vi "Dashboard Main.vi"() -> ()   [LabVIEW 2018]
uses:
  <vilib>/Math Plots/2D Math Plots/2D Compass/2D Compass XCtrl/2D Compass.xctl
  <vilib>/Utility/miscctls.llb/LVRowAndColumnTypeDef.ctl
  <vilib>/event_ctls.llb/eventvkey.ctl
  <vilib>/Rock Robotics/Network Tables/NT Read Numeric Array.vi
  <vilib>/Rock Robotics/Network Tables/NT Write Numeric Array.vi
  <vilib>/Rock Robotics/WPI/Dashboard/WPI_DashboardLogging Global.vi
  <vilib>/Math Plots/2D Math Plots/2D Compass/2D Compass Datatype/2D Compass Datatype.lvclass
  <vilib>/Math Plots/2D Math Plots/2D Compass/2D Compass Datatype/Public/Plot Helper (Vector).vi
  <vilib>/Rock Robotics/Network Tables/NT Read Boolean Array.vi
panel:
  in  "Camera Settings Right":T1={"Frame Rate"=30, "Compression"=30, "Size"=1, "DB Camera Config"=FALSE} {"Frame Rate" scale=1.0..30.0; "Compression" scale=100.0..-1.0; "Size" items=["640x480", "320x240", "160x120"]}
  in  "Camera Name Right":string(combo)="No Camera Selection"
  out "Camera Perf":string
  in  "Camera Settings":T1={"Frame Rate"=30, "Compression"=30, "Size"=1, "DB Camera Config"=FALSE} {"Frame Rate" scale=1.0..30.0; "Compression" scale=100.0..-1.0; "Size" items=["640x480", "320x240", "160x120"]}
  in  "TCP":refnum<k5>
  in  "Rec Mode":enum32{"Stop", "Record", "Playback"}(radio)
  out "Robot IP":string
  out "Image Message":string="Timeout in Camera Communications"
  in  "Dashboard Tab":T2(tab)
  in  "Drive Type":string(combo)
  out "Reversed Modules":bool[](array[boolean])
  out "Front Right Swerve Module":refnum<class "2D Plot Datatype.lvclass">[](xcontrol) caption="2D Compass"
  out "NT Connection":bool
  out "Mode":T3(ring)=enum."Auto Disabled"
  out "Right Camera Perf":cluster{"Bandwidth (Mbps)":dbl, "FPS":dbl}
  in  "Write Swerve Offsets":bool
  out "Back Right Swerve Module":refnum<class "2D Plot Datatype.lvclass">[](xcontrol) caption="2D Compass"
  out "Back Left Swerve Module":refnum<class "2D Plot Datatype.lvclass">[](xcontrol) caption="2D Compass"
  out "Front Left Swerve Module":refnum<class "2D Plot Datatype.lvclass">[](xcontrol) caption="2D Compass"
  out "Scan Radar":picture
  out "Camera Image Right":T4(plugin-control)
  in  "Test Slider":dbl(slide) scale=0.0..100.0 scale format="%#_3g"
  in  "On/Off":bool caption="Solenoid"
  in  "Test Name":u16(ring) items=["Select the test to run..."]
  in  "Test Tree":string(tree)
  in  "Motor":cluster{"Value":dbl, "Enable":bool} {"Value" scale=-1.0..1.0 scale format="%#_3g"}
  out "Progress":T5 {"Test Progress" scale=0.0..100.0}
  in  "Rev/Fwd":cluster{"Forward":bool, "Reverse":bool}
  in  "Test Ring":u16(ring) items=["Monochrome", "Color"]
  out "Cmd Status":string
  in  "Execute Command":bool
  in  "Command Params":string[][](table)
  in  "Command Selection":i32(listbox)
  in  "CheckList":i32(listbox)
  out "Tree":string(tree)
  out "Camera Image":T4(plugin-control)
  out "Background":bool
  in  "Camera Name":string(combo)="No Camera Selection"
  # "HW"
  # "HW"
  # "Drive Options:"
  # "Swerve Vectors:"
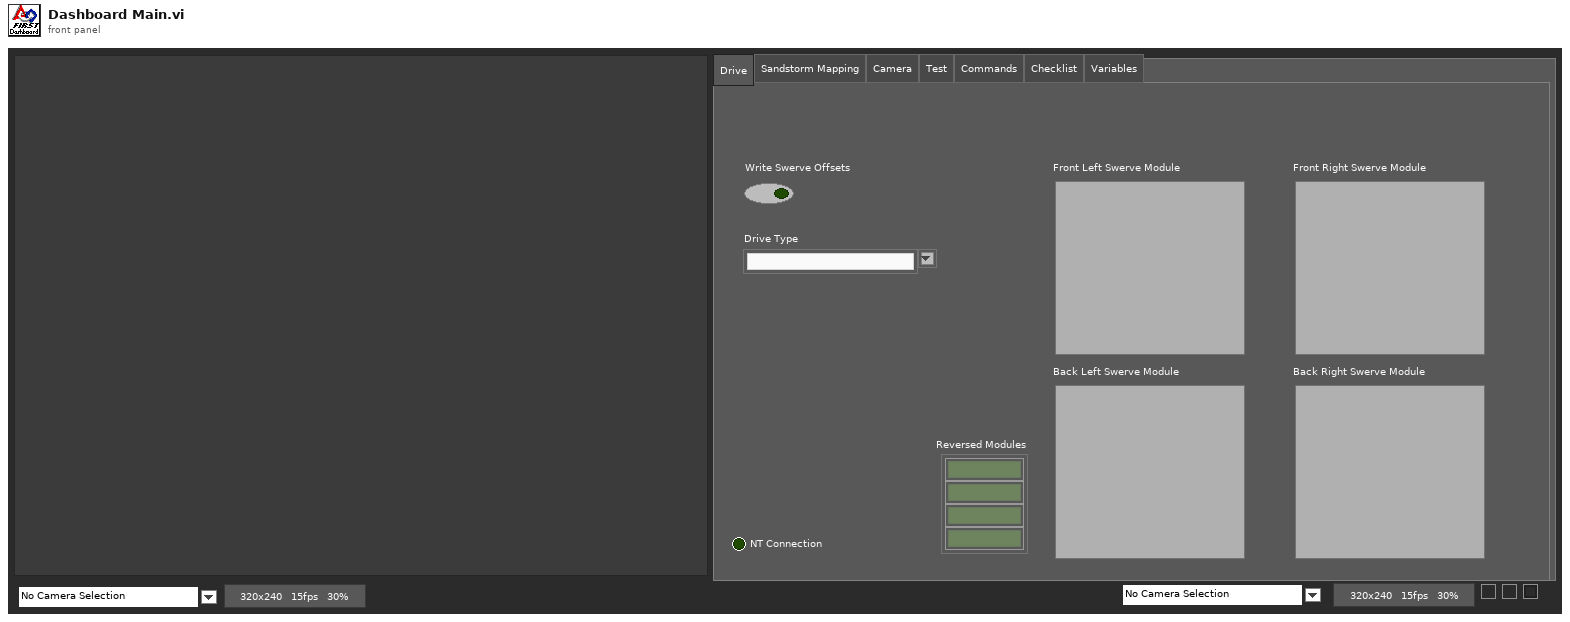
[diagram p1: front panel]
types:
  T1 = cluster{"Frame Rate":i32, "Compression":i32, "Size":u16, "DB Camera Config":bool}
  T2 = enum32{"Drive", "Sandstorm Mapping", "Camera", "Test", "Commands", "Checklist", "Variables"}
  T3 = enum8{"Tele-Op Disabled", "Tele-Op Enabled", "Auto Disabled", "Auto Enabled", "Test Disabled", "Test Enabled", "Disconnected", "No Code", "E-Stop"}
  T4 = typedef "IMAQ Image.ctl" = refnum<image>
  T5 = cluster{"Test Progress":u8, "Test Progress Text":string}
  T6 = cluster{"Save Path":path, "Interval (s)":dbl, "Keep":i32}
  T7 = enum32{"Drive", "Camera", "Basic", "Custom", "Test", "Commands", "Checklist", "Variables"}
  T8 = typedef "Image Type" = u32
  T9 = cluster{"IDs":cluster{"RPC field ID":u16, "Unique ID":u16}, "String":string}
  T10 = enum16{"open", "replace", "create", "open or create", "replace or create", "replace or create with confirmation"}
  T11 = cluster{"Error Strings":string, "Disable Counts":cluster{u16, u16}, "Rail Faults":cluster{u16, u16, u16}, "Robot IP":string, "DB Mode":u8, "Event Info":cluster{"Name":string, "Type":u8, "Number":u16, "Replay":u8}}
  T12 = cluster{"Storage":cluster{"Disk Free":u64, "RAM Block":u32, "RAM free":u32}, "CPU Utilization":cluster{"CPU % ISR":sgl, "CPU % Time Crit":sgl, "CPU % Timed Str":sgl, "CPU % High":sgl, "CPU % Above":sgl, "CPU % Normal":sgl, "CPU % Low":sgl}, "CAN":cluster{"% Bus Utilization":sgl, "Bus Off Cnt":u32, "TX_FIFO Full Cnt":u32, "Receive Error Cnt":u8, "Transmit Error Cnt":u8}, "HID":cluster{"HID Outputs":u32, "Rumble Low":u16, "Rumble High":u16}[]}
  T13 = cluster{"Status bits":cluster{"Test Mode":bool, "Autonomous":bool, "Enabled":bool, "Code Start":bool, "Brownout":bool, "Reserved 2":bool, "Reserved 3":bool, "E-Stop":bool}, "Code Trace":cluster{"Disabled":bool, "TeleOp":bool, "Auto":bool, "Test":bool}, "Controller Type":enum16{"unknown", "cRIO", "roboRio"}, "Code?":enum16{"unknown", "noCode", "code"}, "Battery V":dbl}
  T14 = cluster{"Control Bits":cluster{"TestMode":bool, "Autonomous":bool, "Enabled":bool, "FMS Present":bool, bool, bool, bool, "E-Stop":bool}, "Team Station ":u8, "Countdown":sgl, "Joystick Values":cluster{"Axes":dbl[], "Buttons":bool[], "POVs":i16[]}[]}
  T15 = cluster{"Axes":dbl[], "Buttons":bool[], "POVs":i16[]}[]
  T16 = cluster{"Axes":dbl[], "Buttons":bool[], "POVs":i16[]}
  T17 = typedef "LVBoundsTypeDef.ctl" = cluster{"Width":u32, "Height":u32}
  T18 = cluster{"Camera Image":refnum<vi>, "Dashboard Tab":refnum<vi>, "Background":refnum<vi>, "Rec Mode":refnum<vi>, "Test Slider":refnum<vi>, "On/Off ":refnum<vi>, "Test Ring":refnum<vi>, "Rev/Fwd":refnum<vi>, "Test Name":refnum<vi>, "Motor":refnum<vi>, "Progress":refnum<vi>, "CheckList":refnum<vi>, "Tree":refnum<vi>, "Test Tree":refnum<vi>, "Command Params":refnum<vi>, "Command Selection":refnum<vi>, "Execute Command":refnum<vi>, "Cmd Status":refnum<vi>, "Camera Settings":refnum<vi>, "Camera Name":refnum<vi>, "Camera Perf":refnum<vi>, "Camera Settings Right":refnum<vi>, "Camera Name Right":refnum<vi>, "Camera Image Right":refnum<vi>}
  T19 = cluster{"Global Rectangle":i32[], "Contours":cluster{"Contour Type":u32, "ROI Type":u32, "Points":i32[]}[]}
  T20 = cluster{"Camera Name":string, string, "Saved DB Images Info":cluster{"Save Path":path, "Interval (s)":dbl, "Keep":i32}}
  T21 = cluster{"Camera Name Right":string, string, "Saved DB Images Info":cluster{"Save Path":path, "Interval (s)":dbl, "Keep":i32}}
  T22 = cluster{"Operation":enum16{"Update", "Clear"}, "Color Box":u32}[]
  T23 = typedef "eventvkey.ctl" = enum16{"ASCII", "Enter", "Return", "Shift", "Ctrl", "Alt", "Cmd", "Opt", "Caps", "NumLock", "Clear", "Break", "Up", "Down", "Left", "Right", "Insert", "Delete", "Home", "End", "PageUp", "PageDown", "Escape", "Help", "Pause", "ScrollLock", "F1", "F2", "F3", "F4", "F5", "F6", "F7", "F8", "F9", "F10", "F11", "F12", "F13", "F14", "F15", "F16", "F17", "F18", "F19", "F20", "F21", "F22", "F23", "F24", "Play", "VolumeUp", "VolumeDown", "Mute", "Two Byte Char"}
  T24 = cluster{"Image Size":bool, "Image Type":bool, "Pixel Value":bool, "ROI Information":bool, "Zoom Factor":bool}
  T25 = cluster{"Operation":enum16{"Update", "Clear"}, "Color Box":u32}
  T26 = typedef "LVRowAndColumnTypeDef.ctl" = cluster{"Row":i32, "Column":i32}
  T27 = cluster{"Shift":bool, "Ctrl":bool, "Alt":bool, "Cmd":bool, "Opt":bool}
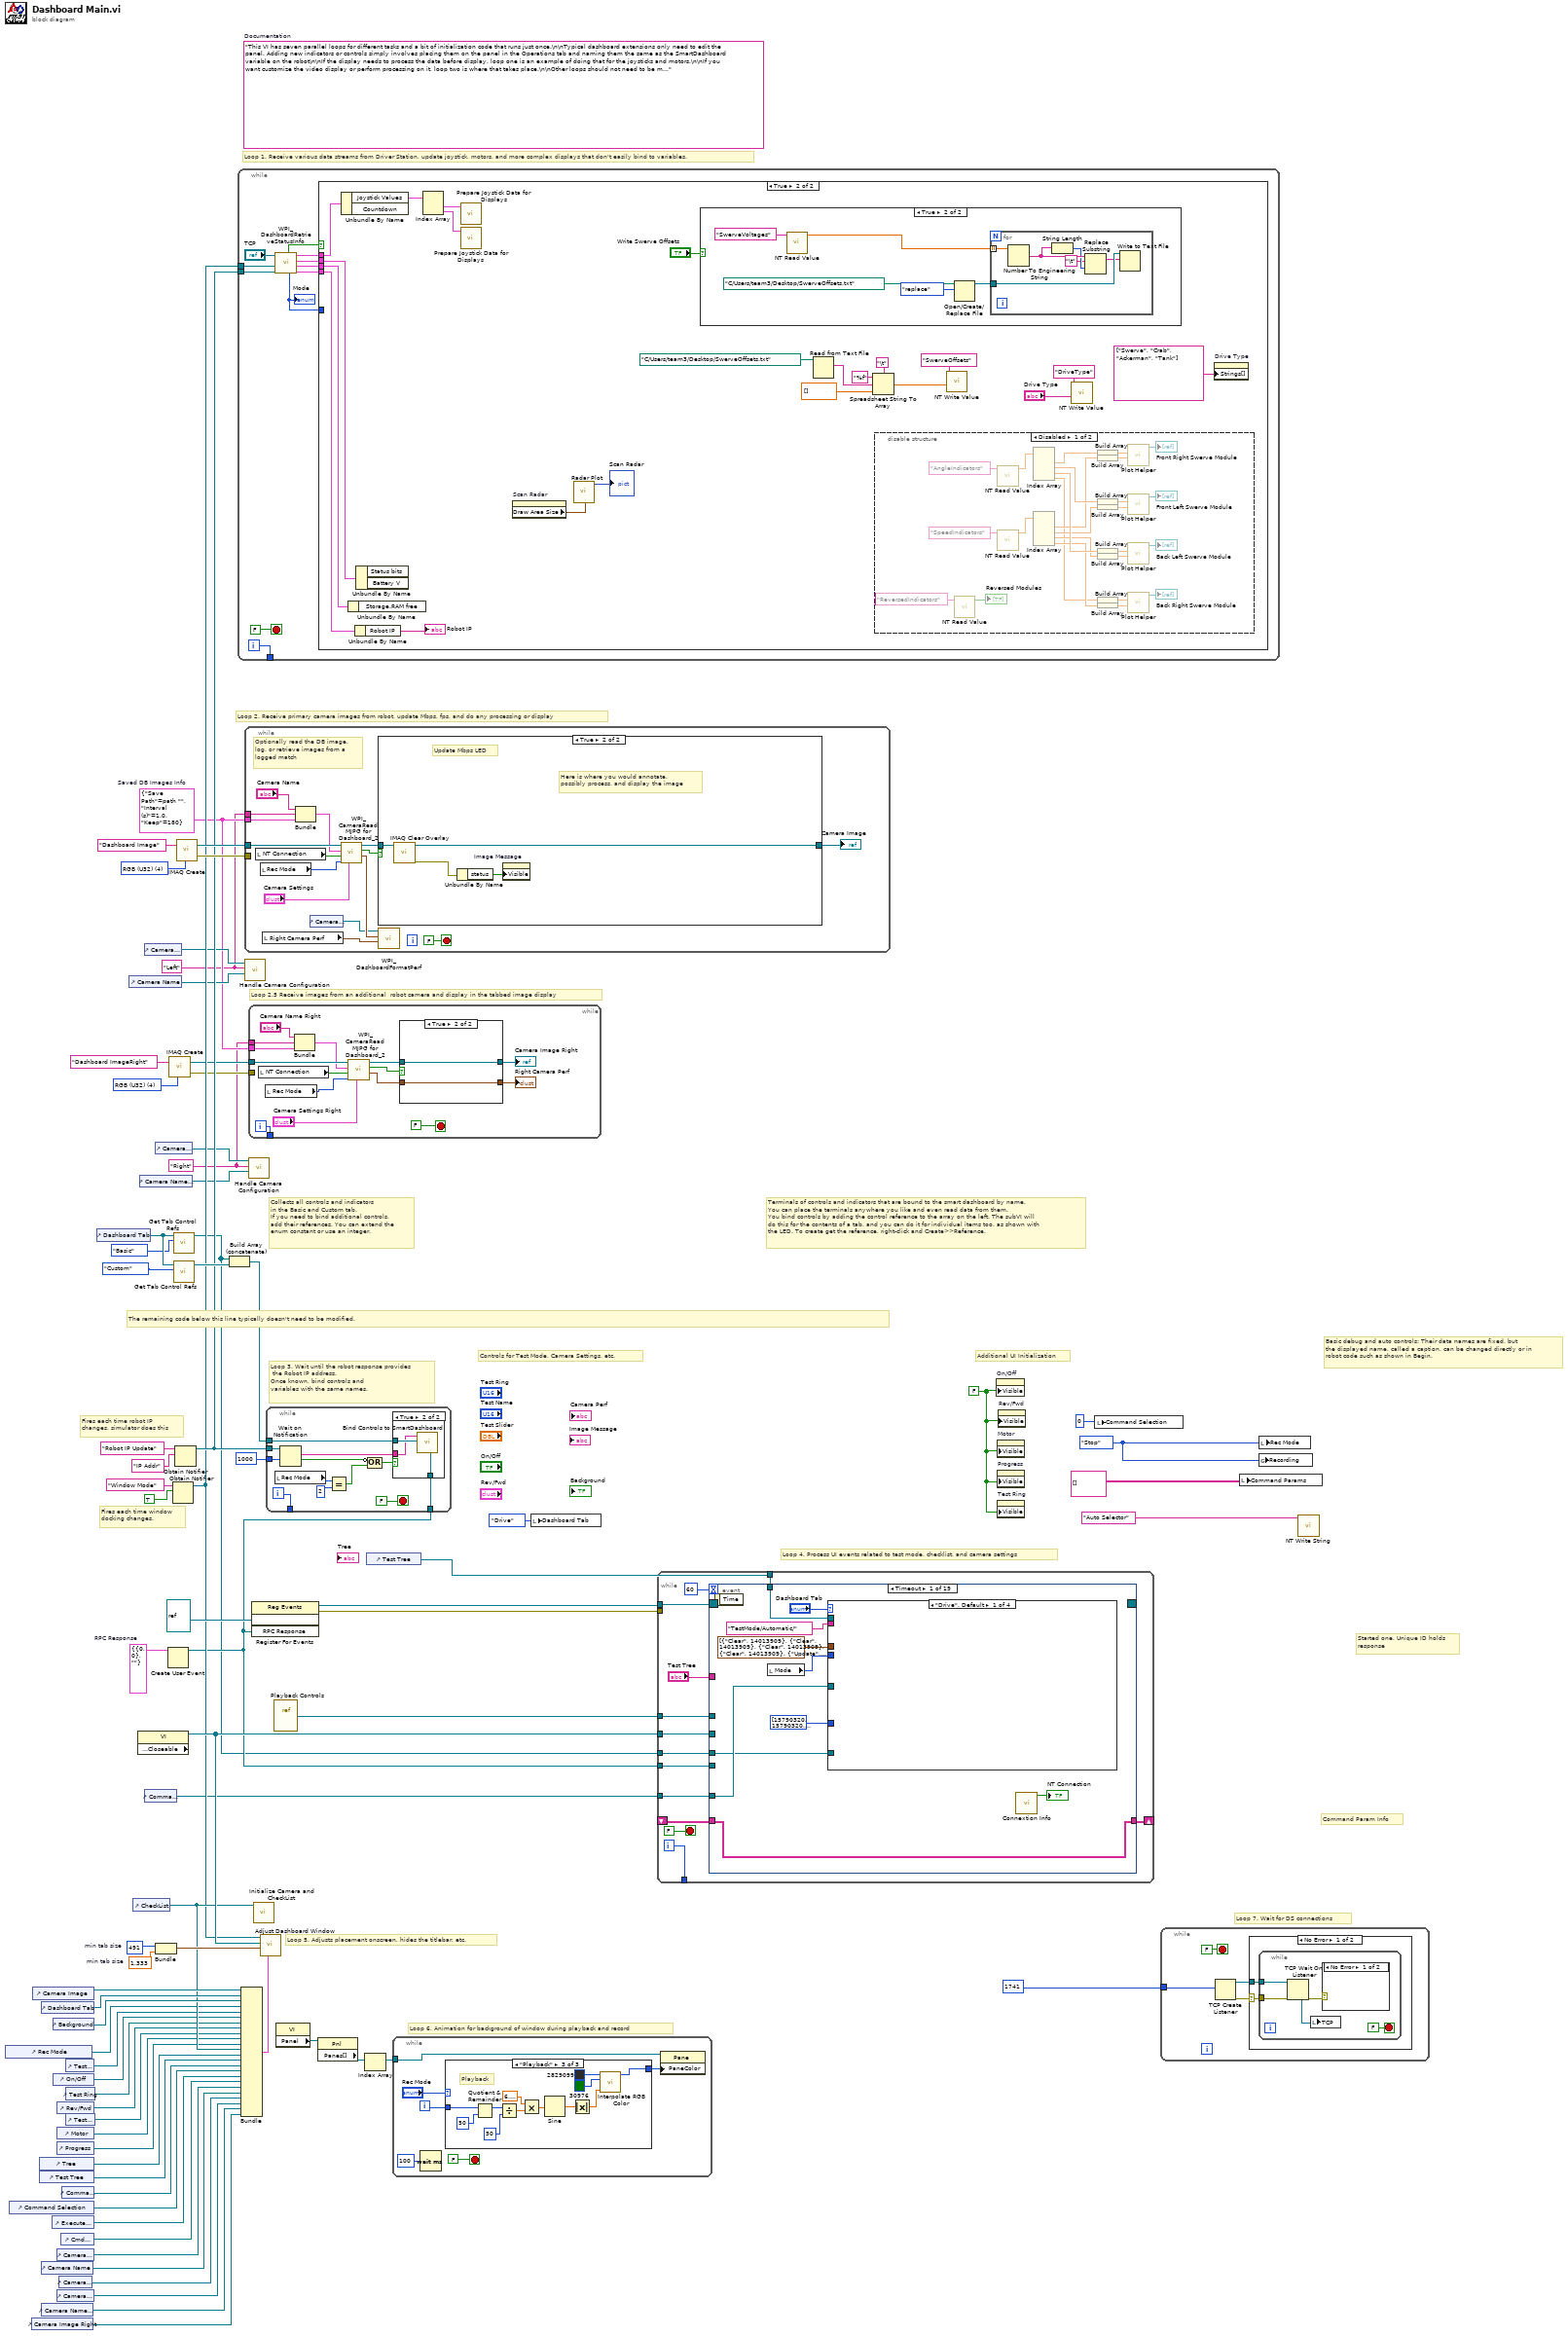
[diagram p0: block diagram]
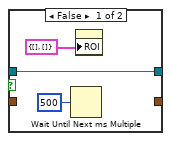
[diagram p2: hidden frame]
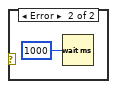
[diagram p3: hidden frame]
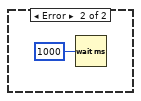
[diagram p4: hidden frame]
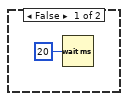
[diagram p5: hidden frame]
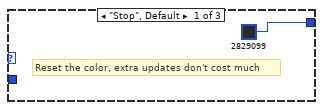
[diagram p8: hidden frame]
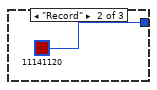
[diagram p9: hidden frame]
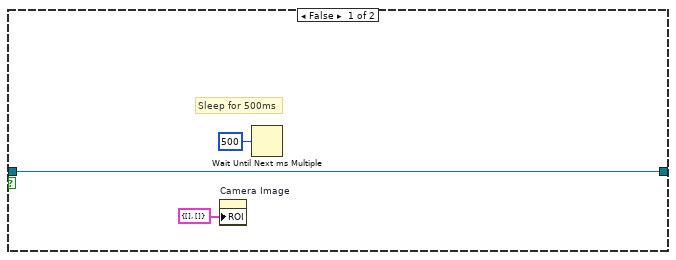
[diagram p11: hidden frame]
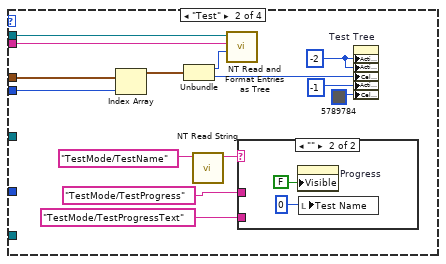
[diagram p12: hidden frame]
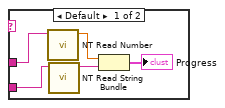
[diagram p13: hidden frame]
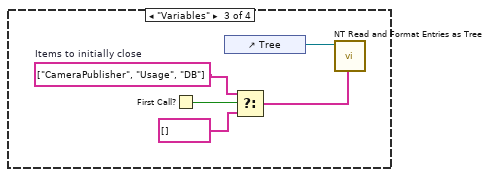
[diagram p14: hidden frame]
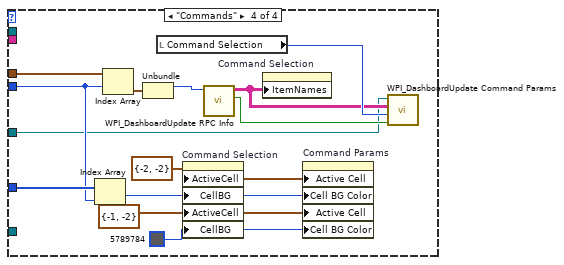
[diagram p15: hidden frame]
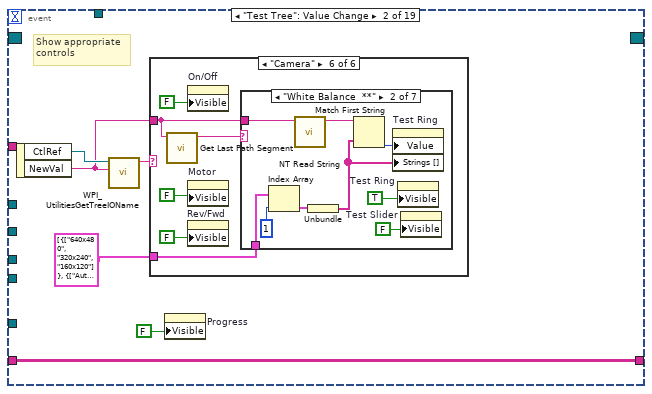
[diagram p16: hidden frame]
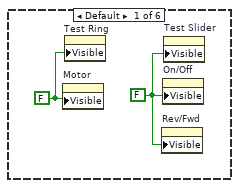
[diagram p17: hidden frame]
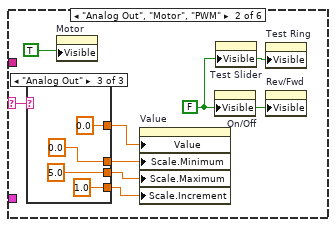
[diagram p18: hidden frame]
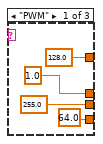
[diagram p19: hidden frame]
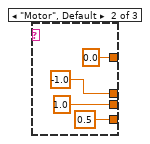
[diagram p20: hidden frame]
diagram:
  w4 = T6 {"Save Path"=path "", "Interval (s)"=1.0, "Keep"=180}  # Saved DB Images Info
  w3 = "Right"
  w2 = "Left"
  w14 = T8 4 items=["Grayscale (U8)", "Grayscale (I16)", "Grayscale (SGL)", "Complex (CSG)", "RGB (U32)", "HSL (U32)", "RGB (U64)"] ("Image Type")
  w29 = T9 {"IDs"={"RPC field ID"=0, "Unique ID"=0}, "String"=""}  # RPC Response
  w51 = 491  # min tab size
  w50 = 1.333  # min tab size
  w58 = enum32{"Stop", "Record", "Playback"}."Stop" ("Rec Mode")
  w35 = FALSE ("Visible")
  (unwired) "This VI has seven parallel loops for different tasks and a bit of initialization code that runs just once.\n\nTypical dashboard extensions only need to edit the panel. Adding new indicators or controls simply involves placing them on the panel in the Operations tab and naming them the same as the SmartDashboard variable on the robot\n\nIf the display needs to process the data before display, loop one is an example of doing that for the joysticks and motors.\n\nIf you want customize the video display or perform processing on it, loop two is where that takes place.\n\nOther loops should not need to be modified. They are pretty standard, and document the task they perform."  # Documentation
  w75 = T8 4 items=["Grayscale (U8)", "Grayscale (I16)", "Grayscale (SGL)", "Complex (CSG)", "RGB (U32)", "HSL (U32)", "RGB (U64)"] ("Image Type")
  # "Loop 2.5 Receive images from an additional  robot camera and display in the tabbed image display"
  # "Command Param Info"
  # "Started one, Unique ID holds\nresponse"
  # "Loop 7. Wait for DS connections"
  # "Basic debug and auto controls: Their data names are fixed, but\nthe displayed name, called a caption, can be changed directly or in\nrobot code such as shown in Begin."
  # "Controls for Test Mode, Camera Settings, etc."
  # "Additional UI Initialization"
  # "Loop 6. Animation for background of window during playback and record"
  # "Fires each time robot IP\nchanges, simulator does this"
  # "Fires each time window\ndocking changes."
  # "Collects all controls and indicators\nin the Basic and Custom tab.\nIf you need to bind additional controls,\nadd their references. You can extend the\nenum constant or use an integer."
  # "The remaining code below this line typically doesn't need to be modified."
  # "Loop 4. Process UI events related to test mode, checklist, and camera settings"
  # "Terminals of controls and indicators that are bound to the smart dashboard by name.\nYou can place the terminals anywhere you like and even read data from them.\nYou bind controls by adding the control reference to the array on the left. The subVI will\ndo this for the contents of a tab, and you can do it for individual items too, as shown with\nthe LED. To create get the reference, right-click and Create>>Reference."
  # "Loop 3. Wait until the robot response provides\n the Robot IP address.\nOnce known, bind controls and\nvariables with the same names."
  # "Loop 5. Adjusts placement onscreen, hides the titlebar, etc."
  # "Loop 1. Receive various data streams from Driver Station, update joystick, motors, and more complex displays that don't easily bind to variables."
  # "Loop 2. Receive primary camera images from robot, update Mbps, fps, and do any processing or display"
  n1 = control-ref of="Rec Mode"() -> (w41:refnum<vi>)
  n2 = control-ref of="Command Selection"() -> (w28:refnum<vi>)
  n3 = control-ref of="Camera Image Right"() -> (w7:refnum<vi>)
  n4 = control-ref of="Camera Image"() -> (w53:refnum<vi>)
  n5 = control-ref of="Tree"() -> (w45:refnum<vi>)
  n6 = control-ref of="Test Tree"() -> (w44:refnum<vi>)
  n7 = control-ref of="Dashboard Tab"() -> (w52:refnum<vi>)
  n8 = control-ref of="Camera Name"() -> (w19:refnum<vi>)
  n9 = control-ref of="Camera Name Right"() -> (w8:refnum<vi>)
  n10 = control-ref of="Execute Command"() -> (w30:refnum<vi>)
  n11 = control-ref of="Background"() -> (w48:refnum<vi>)
  n12 = control-ref of="On/Off"() -> (w39:refnum<vi>)
  n13 = control-ref of="Progress"() -> (w36:refnum<vi>)
  n14 = control-ref of="Camera Settings"() -> (w20:refnum<vi>)
  n15 = control-ref of="Camera Settings Right"() -> (w9:refnum<vi>)
  n16 = control-ref of="Rev/Fwd"() -> (w37:refnum<vi>)
  n17 = control-ref of="Motor"() -> (w42:refnum<vi>)
  n18 = control-ref of="Camera Perf"() -> (w18:refnum<vi>)
  n19 = control-ref of="Cmd Status"() -> (w24:refnum<vi>)
  n20 = control-ref of="Command Params"() -> (w31:refnum<vi>)
  n21 = control-ref of="Test Slider"() -> (w40:refnum<vi>)
  n22 = control-ref of="Test Ring"() -> (w38:refnum<vi>)
  n23 = control-ref of="Test Name"() -> (w43:refnum<vi>)
  n24 = control-ref of="Dashboard Tab"() -> (w56:refnum<vi>)
  n25 = control-ref of="Camera Name"() -> (w21:refnum<vi>)
  n26 = control-ref of="CheckList"() -> (w46:refnum<vi>)
  n27 = property class="VI" props=["Front Panel.Closeable"]() -> (reference out=w57:refnum<vi>)  [unwired: 2 in, 2 out]
  n28 = control-ref of="Camera Name Right"() -> (w10:refnum<vi>)
  n29 = control-ref of="Camera Settings"() -> (w22:refnum<vi>)
  n30 = control-ref of="Command Params"() -> (w23:refnum<vi>)
  n31 = control-ref of="Camera Settings Right"() -> (w11:refnum<vi>)
  n32 = Bundle("min tab size"=w51, "min tab size"=w50) -> (w49:cluster{"min tab size":i32, "min tab size":dbl})  [unwired: 1 in]
  n33 = Create User Event(user event datatype=w29) -> (user event=w25:refnum<user-event>)  [unwired: 1 in, 1 out]
  n34 = call "IMAQ Create"("Image Name"="Dashboard ImageRight", "Image Type"=w14) -> ("New Image"=w13:T4, "error out"=w12:errorcluster)  [unwired: 2 in, 1 out]
  n35 = Obtain Notifier(name (unnamed)="Window Mode", notification data type=TRUE) -> (notifier out=w33:refnum<notifier>)  [unwired: 2 in, 2 out]
  n36 = call <vilib>:"Get Tab Control Refs.vi"("Page Index"=T7."Basic" ("Dashboard Tab"), "TabControl in"=w56) -> ("ControlsOnPage"=w17:refnum<vi>[])  [unwired: 9 in]
  n37 = call <vilib>:"Get Tab Control Refs.vi"("Page Index"=T7."Custom" ("Dashboard Tab"), "TabControl in"=w56) -> ("ControlsOnPage"=w55:refnum<vi>[])  [unwired: 9 in]
  n38 = Obtain Notifier(name (unnamed)="Robot IP Update", notification data type="IP Addr" ("name (unnamed)")) -> (notifier out=w34:refnum<notifier>)  [unwired: 2 in, 2 out]
  n39 = call "IMAQ Create"("Image Name"="Dashboard Image", "Image Type"=w75) -> ("New Image"=w73:T4, "error out"=w72:errorcluster)  [unwired: 2 in, 1 out]
  n40 = Build Array (concatenate)(w17, w55) -> (w54:refnum<vi>[])
  n41 = while {
    tunnel: [w85] -> _
    tunnel: w34 -> [w79]
    tunnel: w33 -> [w76]
    i -> [w85]
    stop <- FALSE stop-if-true
    n42 = call <vilib>:"WPI_DashboardRetrieveStatusInfo.vi"("Binding Refnum"=w79, "Window Mode Notifier"=w76, "TCP Cnx"="TCP") -> ("Power and Errors"=w80:T11, "Robot Metrics"=w83:T12, "Status Info"=w84:T13, "Control Info"=w81:T14, "Robot Mode"=w78:T3, "Process?"=w82:bool)  [unwired: 3 in]
    "Mode" <- w78
    n43 = case shown="True" w82 {
      tunnel: w84 -> [_ w108]
      tunnel: w83 -> [_ w107]
      tunnel: w81 -> [_ w106]
      tunnel: w80 -> [_ w105]
      tunnel: w78 -> [_ _]
      frame False {
        n44 = Wait (ms)(milliseconds to wait=u32 20) -> ()  [unwired: 1 out]
      }
      frame True {
        n45 = Unbundle By Name(w106) -> ("Joystick Values"=w99:T15)  [unwired: 1 out]
        n46 = Unbundle By Name(w107) -> ()  [unwired: 1 out]
        n47 = Unbundle By Name(w105) -> ("Robot IP"=→"Robot IP":string)
        n48 = Unbundle By Name(w108) -> ()  [unwired: 2 out]
        n49 = Index Array(array=w99) -> (element #1=w104:T16, element #2=w103:T16)  [unwired: 2 in]
        n50 = call "Prepare Joystick Data for Displays.vi"("Joystick Values"=w104) -> ()  [unwired: 8 in, 3 out]
        n51 = call "Prepare Joystick Data for Displays.vi"("Joystick Values"=w103) -> ()  [unwired: 8 in, 3 out]
        n52 = property on="Scan Radar" class="Pict"() -> ("Draw Area Size"=w97:T17)  [unwired: 2 in, 2 out]
        n53 = call <vilib>:"Radar Plot.vi"("dimension (w,h)"=w97) -> ("new picture"=→"Scan Radar":picture)  [unwired: 14 in]
        n54 = case shown="True" "Write Swerve Offsets" {
          frame False {
          }
          frame True {
            n55 = call-poly <vilib>:"NT Read Value.vi"("Name"="SwerveVoltages") -> ("Numeric Array"=w135:dbl[])  [unwired: 9 in, 1 out]
            n56 = Open/Create/Replace File(file path (use dialog)=path "C:/Users/team3/Desktop/SwerveOffsets.txt" ("file (use dialog)"), operation (0:open)=T10."replace") -> (refnum out=w138:refnum<file>)  [unwired: 4 in, 2 out]
            n57 = for {
              tunnel: w138 -> [w144]
              tunnel: w135 -> [w145] mode=indexing
              n58 = Number To Engineering String(4:w145) -> (0:w143:string)  [unwired: 3 in]
              n59 = String Length(string=w143) -> (length=w142:i32)
              n60 = Replace Substring(3:w142, 4:"\t", 5:w143) -> (1:w140:string)  [unwired: 1 in, 1 out]
              n61 = Write to Text File(file (use dialog)=w144, text=w140) -> ()  [unwired: 2 in, 3 out]
            }
          }
        }
        n62 = Read from Text File(file (use dialog)=path "C:/Users/team3/Desktop/SwerveOffsets.txt") -> (text=w92:string)  [unwired: 3 in, 3 out]
        n63 = Spreadsheet String To Array(delimiter (Tab)="\t", format string="%f", spreadsheet string=w92, array type (2D Dbl)=dbl[] []) -> (array=w91:dbl[])
        n64 = disable-structure shown="Disabled" {
          frame Disabled {
            n65 = call-poly <vilib>:"NT Read Value.vi"("Name"="ReversedIndicators") -> ("Boolean Array"=→"Reversed Modules":bool[])  [unwired: 9 in, 1 out]
            n66 = call-poly <vilib>:"NT Read Value.vi"("Name"="AngleIndicators") -> ("Numeric Array"=w127:dbl[])  [unwired: 9 in, 1 out]
            n67 = call-poly <vilib>:"NT Read Value.vi"("Name"="SpeedIndicators") -> ("Numeric Array"=w126:dbl[])  [unwired: 9 in, 1 out]
            n68 = Index Array(array=w127) -> (element #1=w122:dbl, element #2=w121:dbl, element #3=w120:dbl, element #4=w109:dbl)  [unwired: 4 in]
            n69 = Index Array(array=w126) -> (element #1=w117:dbl, element #2=w114:dbl, element #3=w112:dbl, element #4=w110:dbl)  [unwired: 4 in]
            n70 = Build Array(w122) -> (w124:dbl[])
            n71 = Build Array(w117) -> (w116:dbl[])
            n72 = Build Array(w121) -> (w123:dbl[])
            n73 = Build Array(w114) -> (w115:dbl[])
            n74 = Build Array(w120) -> (w119:dbl[])
            n75 = Build Array(w112) -> (w113:dbl[])
            n76 = Build Array(w109) -> (w118:dbl[])
            n77 = Build Array(w110) -> (w111:dbl[])
            n78 = call-poly <vilib>:"Plot Helper.vi"("radius vector"=w116, "theta vector"=w124) -> ("2D Plot Class Obj Array out"=→"Front Right Swerve Module":refnum<class "2D Plot Datatype.lvclass">[])  [unwired: 2 in, 7 out]
            n79 = call-poly <vilib>:"Plot Helper.vi"("radius vector"=w115, "theta vector"=w123) -> ("2D Plot Class Obj Array out"=→"Front Left Swerve Module":refnum<class "2D Plot Datatype.lvclass">[])  [unwired: 2 in, 7 out]
            n80 = call-poly <vilib>:"Plot Helper.vi"("radius vector"=w113, "theta vector"=w119) -> ("2D Plot Class Obj Array out"=→"Back Left Swerve Module":refnum<class "2D Plot Datatype.lvclass">[])  [unwired: 2 in, 7 out]
            n81 = call-poly <vilib>:"Plot Helper.vi"("radius vector"=w111, "theta vector"=w118) -> ("2D Plot Class Obj Array out"=→"Back Right Swerve Module":refnum<class "2D Plot Datatype.lvclass">[])  [unwired: 2 in, 7 out]
          }
          frame Enabled {
          }
        }
        n82 = call-poly <vilib>:"NT Write Value.vi"("Numeric Array"=w91, "Name"="SwerveOffsets") -> ()  [unwired: 9 in, 1 out]
        n83 = call-poly <vilib>:"NT Write Value.vi"("String"="Drive Type", "Name"="DriveType") -> ()  [unwired: 9 in, 1 out]
        n84 = property on="Drive Type" class="CmbBox"("Strings[]"=string[] ["Swerve", "Crab", "Ackerman", "Tank"] ("Strings []")) -> ()  [unwired: 2 in, 2 out]
      }
    }
  }
  n85 = Bundle("Camera Image"=w53, "Dashboard Tab"=w52, "Background"=w48, "Rec Mode"=w41, "Test Slider"=w40, "On/Off"=w39, "Test Ring"=w38, "Rev/Fwd"=w37, "Test Name"=w43, "Motor"=w42, "Progress"=w36, "CheckList"=w46, "Tree"=w45, "Test Tree"=w44, "Command Params"=w31, "Command Selection"=w28, "Execute Command"=w30, "Cmd Status"=w24, "Camera Settings"=w20, "Camera Name"=w19, "Camera Perf"=w18, "Camera Settings Right"=w9, "Camera Name Right"=w8, "Camera Image Right"=w7) -> (w47:T18)  [unwired: 1 in]
  n86 = call "Handle Camera Configuration.vi"("CameraNameRef"=w21, "Display Name"=w2, "ClusterRef"=w22) -> ()  [unwired: 9 in]
  n87 = while {
    tunnel: w73 -> [w159]
    tunnel: w72 -> [_]
    tunnel: w4 -> [w152]
    tunnel: w2 -> [w149]
    stop <- FALSE stop-if-true
    # "Optionally read the DB image,\nlog, or retrieve images from a\nlogged match"
    n88 = local read "NT Connection"() -> (w153:bool)
    n89 = local read "Rec Mode"() -> (w156:enum32{"Stop", "Record", "Playback"})
    n90 = local read "Right Camera Perf"() -> (w147:cluster{"Bandwidth (Mbps)":dbl, "FPS":dbl})
    n91 = Bundle("Camera Name"="Camera Name", w149, "Saved DB Images Info"=w152) -> (w151:T20)  [unwired: 1 in]
    n92 = control-ref of="Camera Perf"() -> (w146:refnum<vi>)
    n93 = call <vilib>:"WPI_CameraRead MJPG for Dashboard_2.vi"("Camera Settings"="Camera Settings", "Rec Mode"=w156, "NT Connection"=w153, "Capture Info"=w151, "Image in"=w159) -> ("perf info"=w148:cluster{"Bandwidth (Mbps)":dbl, "fps":dbl}, "Active"=w157:bool, "Image\\ out"=w158:T4)  [unwired: 4 in]
    n94 = case shown="True" w157 {
      tunnel: w158 -> [w162 w165]
      tunnel: [w162 w164] -> w154
      frame False {
        # "Sleep for 500ms"
        n95 = property on="Camera Image" class="ImageControl"("ROI"=T19 {"Global Rectangle"=[], "Contours"=[]}) -> ()  [unwired: 2 in, 2 out]
        n96 = Wait Until Next ms Multiple(millisecond multiple=u32 500) -> ()  [unwired: 1 out]
      }
      frame True {
        # "Here is where you would annotate,\npossibly process, and display the image"
        # "Update Mbps LED"
        n97 = call "IMAQ Clear Overlay"("Image"=w165) -> ("error out"=w166:errorcluster, "Image Out"=w164:T4)  [unwired: 2 in, 7 out]
        n98 = Unbundle By Name(w166) -> ("status"=w167:bool)
        n99 = property on="Image Message" class="Str"("Visible"=w167) -> ()  [unwired: 2 in, 2 out]
      }
    }
    "Camera Image" <- w154
    n100 = call <vilib>:"WPI_DashboardFormatPerf.vi"("Right Camera Perf"=w147, "Performance"=w148, "String in"=w146) -> ()  [unwired: 9 in]
  }
  n101 = call "Handle Camera Configuration.vi"("CameraNameRef"=w10, "Display Name"=w3, "ClusterRef"=w11) -> ()  [unwired: 9 in]
  n102 = while {
    tunnel: w13 -> [w182]
    tunnel: w12 -> [_]
    tunnel: [w177] -> _
    tunnel: w4 -> [w173]
    tunnel: w3 -> [w170]
    i -> [w177]
    stop <- FALSE stop-if-true
    n103 = local read "NT Connection"() -> (w174:bool)
    n104 = local read "Rec Mode"() -> (w181:enum32{"Stop", "Record", "Playback"})
    n105 = Bundle("Camera Name Right"="Camera Name Right", w170, "Saved DB Images Info"=w173) -> (w172:T21)  [unwired: 1 in]
    n106 = call <vilib>:"WPI_CameraRead MJPG for Dashboard_2.vi"("Camera Settings"="Camera Settings Right", "Rec Mode"=w181, "NT Connection"=w174, "Capture Info"=w172, "Image in"=w182) -> ("perf info"=w168:cluster{"Bandwidth (Mbps)":dbl, "fps":dbl}, "Active"=w176:bool, "Image\\ out"=w179:T4)  [unwired: 4 in]
    n107 = case shown="True" w176 {
      tunnel: w179 -> [w184 w187]
      tunnel: [w184 w187] -> w175
      tunnel: [_ w186] -> w169
      tunnel: w168 -> [_ w186]
      frame False {
        n108 = Wait Until Next ms Multiple(millisecond multiple=u32 500) -> ()  [unwired: 1 out]
        n109 = property on="Camera Image Right" class="ImageControl"("ROI"=T19 {"Global Rectangle"=[], "Contours"=[]}) -> ()  [unwired: 2 in, 2 out]
      }
      frame True {
      }
    }
    "Camera Image Right" <- w175
    "Right Camera Perf" <- w169
  }
  n110 = register-events(refnum<vi> refnum, w25) -> (reference out=w62:refnum<event-registration>, error out=w61:errorcluster)  [unwired: 2 in]
  n111 = call "Initialize Camera and CheckList.vi"("ListBox in"=w46) -> ()  [unwired: 11 in]
  n112 = call "Adjust Dashboard Window.vi"("Sizing Refnums"=w47, "Size Constraints"=w49, "VI"=w57, "WIn Mode"=w33) -> ()  [unwired: 8 in]
  n113 = while {
    tunnel: w54 -> [w199]
    tunnel: w34 -> [w197]
    tunnel: [w195] -> _
    tunnel: u32 1000 ("milliseconds to wait") -> [w194]
    tunnel: w25 -> [w188]
    i -> [w195]
    stop <- FALSE stop-if-true
    n114 = local read "Rec Mode"() -> (w190:enum32{"Stop", "Record", "Playback"})
    n115 = Wait on Notification(notifier=w197, timeout in ms (-1)=w194) -> (notification=w196:string, timed out?=w192:bool)  [unwired: 2 in, 2 out]
    n116 = Equal?(x=w190, y=u16 2 ("Rec Mode")) -> (x = y?=w191:bool)
    n117 = Compound Arithmetic op=OR(invert w192, w191) -> (w193:bool)
    n118 = case shown="True" w193 {
      tunnel: w199 -> [_ w202]
      tunnel: w196 -> [_ w201]
      tunnel: w188 -> [_ w200]
      frame False {
      }
      frame True {
        n119 = call <vilib>:"Bind Controls to SmartDashboard.vi"("RPC ref"=w200, "Bound Control Refs"=w202, "Server IP Address"=w201) -> ()  [unwired: 9 in]
      }
    }
  }
  n120 = vi-ref "Playback Controls.vi"() -> (w63:refnum<vi>)
  n121 = property class="VI"() -> ("Panel"=w65:refnum<vi>)  [unwired: 2 in, 2 out]
  n122 = property class="Pnl"(reference=w65) -> ("Panes[]"=w66:refnum<vi>[])  [unwired: 1 in, 2 out]
  n123 = Index Array(array=w66) -> (element=w64:refnum<vi>)  [unwired: 1 in]
  n124 = control-ref of="Test Tree"() -> (w67:refnum<vi>)
  n125 = while {
    tunnel: w64 -> [w204]
    i -> [w207]
    stop <- FALSE stop-if-true
    n126 = Wait (ms)(milliseconds to wait=u32 100) -> ()  [unwired: 1 out]
    n127 = case shown="\"Playback\"" "Rec Mode" {
      tunnel: w207 -> [_ _ w222]
      tunnel: [u32 2829099 ("Base Color") u32 11141120 ("Target Color") w211] -> w203
      frame "Stop", Default {
        # "Reset the color, extra updates don't cost much"
      }
      frame "Record" {
      }
      frame "Playback" {
        # "Playback"
        n128 = Quotient & Remainder(x=w222, y=u32 50 ("milliseconds to wait")) -> (x-y*floor(x/y)=w218:u32)  [unwired: 1 out]
        n129 = Divide(x=w218, y=u32 50 ("milliseconds to wait")) -> (x/y=w215:dbl)
        n130 = Multiply(x=6.283185307179586, y=w215) -> (x*y=w220:dbl)
        n131 = Sine(x=w220) -> (sin(x)=w219:dbl)
        n132 = Absolute Value(x=w219) -> (abs(x)=w212:dbl)
        n133 = call "Interpolate RGB Color.vi"("Proportion"=w212, "Target Color"=u32 30976, "Base Color"=u32 2829099) -> ("Result Color"=w211:u32)  [unwired: 8 in]
      }
    }
    n134 = property class="Pane"(reference=w204, "PaneColor"=w203) -> ()  [unwired: 1 in, 2 out]
  }
  n135 = local write "Dashboard Tab"(T2."Drive" ("Dashboard Tab")) -> ()
  n136 = while {
    tunnel: [w232] -> _
    tunnel: w67 -> [w231]
    tunnel: w63 -> [w230]
    tunnel: w62 -> [w229]
    tunnel: w61 -> [_]
    tunnel: w57 -> [w228]
    tunnel: w25 -> [w227]
    tunnel: w23 -> [w226]
    shift-right: [w225] -> _
    shift-left: _ -> [w224]
    tunnel: w17 -> [w223]
    i -> [w232]
    stop <- FALSE stop-if-true
    n137 = event shown="[0] Timeout" {
      selector: w229 -> [_ _ _ _ _ _ _ _ _ _ _ _ _ _ _ _ _ _ _]
      dyn-events: [_ _ _ _ _ _ _ _ _ _ _ _ _ _ w485 _ _ _ _] -> _
      timeout: u32 60 ("milliseconds to wait") -> [_ _ _ _ _ _ _ _ _ _ _ _ _ _ _ _ _ _ _]
      tunnel: w231 -> [w244 _ _ _ _ _ _ _ _ _ _ _ _ _ _ _ _ _ _]
      tunnel: "Test Tree" -> [_ _ _ _ _ _ _ _ _ w452 w460 w462 w466 w474 _ _ _ _ _]
      tunnel: w230 -> [_ _ _ _ _ _ _ _ _ _ _ _ _ _ w487 _ w505 _ _]
      tunnel: w228 -> [_ _ _ _ _ _ _ _ _ _ _ _ _ _ w483 _ _ _ _]
      tunnel: w227 -> [_ _ _ _ _ _ _ _ _ _ _ _ _ _ w481 _ _ _ _]
      tunnel: w226 -> [w239 _ _ _ w403 _ _ _ _ _ _ _ _ _ _ _ _ _ _]
      tunnel: [w238 w286 w388 w393 w401 w410 w420 w427 w439 w451 w458 w461 w465 w473 w480 w500 w502 w506 w519] -> w225
      tunnel: w224 -> [w238 w286 w388 w393 w401 _ _ w427 w439 w451 w458 w461 w465 w473 w480 w500 w502 w506 w519]
      tunnel: w223 -> [w236 _ _ _ _ _ _ _ _ _ _ _ _ _ _ _ _ _ _]
      event Timeout {
        n138 = event-data() -> ()  [unwired: 1 in, 1 out]
        n139 = local read "Mode"() -> (w241:T3)
        n140 = case shown="\"Drive\", Default" "Dashboard Tab" {
          tunnel: w244 -> [_ w259 _ _]
          tunnel: "TestMode/Automatic/" ("Name Pattern") -> [_ w258 _ _]
          tunnel: T22 [{"Operation"=enum."Clear", "Color Box"=14013909}, {"Operation"=enum."Clear", "Color Box"=14013909}, {"Operation"=enum."Clear", "Color Box"=14013909}, {"Operation"=enum."Clear", "Color Box"=14013909}, {"Operation"=enum."Update", "Color Box"=14013909}, {"Operation"=enum."Update", "Color Box"=16777215}, {"Operation"=enum."Clear", "Color Box"=14013909}, {"Operation"=enum."Clear", "Color Box"=14013909}, {"Operation"=enum."Clear", "Color Box"=14013909}] -> [_ w251 _ w279]
          tunnel: w241 -> [_ w250 _ w278]
          tunnel: u32[] [15790320, 15790320, 15790320, 15790320, 16777215, 16777215, 15790320, 15790320, 15790320] -> [_ _ _ w284]
          tunnel: w239 -> [_ _ _ w272]
          tunnel: w236 -> [_ _ _ _]
          frame "Drive", Default {
          }
          frame "Test" {
            w257 = -2 ("Active Item:Row Number")
            n141 = Index Array(array=w251, index=w250) -> (element=w252:T25)
            n142 = Unbundle(w252) -> ("Operation"=w253:enum16{"Update", "Clear"}, "Color Box"=w254:u32)
            n143 = call <vilib>:"NT Read String.vi"("Name"="TestMode/TestName") -> ("String"=w248:string)  [unwired: 9 in, 1 out]
            n144 = call <vilib>:"NT Read and Format Entries as Tree.vi"("Operation"=w253, "Name Pattern"=w258, "Tree Refnum"=w259) -> ()  [unwired: 7 in, 2 out]
            n145 = case shown="\"\"" w248 {
              tunnel: "TestMode/TestProgress" ("Name") -> [w261 _]
              tunnel: "TestMode/TestProgressText" ("Name") -> [w260 _]
              frame Default {
                n146 = call <vilib>:"NT Read Number.vi"("Name"=w261) -> ("Numeric"=w262:dbl)  [unwired: 9 in, 1 out]
                n147 = call <vilib>:"NT Read String.vi"("Name"=w260) -> ("String"=w263:string)  [unwired: 9 in, 1 out]
                n148 = Bundle("Numeric"=w262, "String"=w263) -> (→"Progress":cluster{"Numeric":dbl, "String":string})  [unwired: 1 in]
              }
              frame "" {
                n149 = property on="Progress" class="Clust (strict)"("Visible"=FALSE) -> ()  [unwired: 2 in, 2 out]
                n150 = local write "Test Name"(u16 0) -> ()
              }
            }
            n151 = property on="Test Tree" class="Tree (strict)"("Active Item Row Number"=w257, "ActiveColNum"=w257, "CellBG"=w254, "Active Item Row Number"=-1 ("Active Item:Row Number"), "CellBG"=u32 5789784 ("Color Box")) -> ()  [unwired: 2 in, 2 out]
          }
          frame "Variables" {
            w269 = string[] ["CameraPublisher", "Usage", "DB"]  # Items to initially close
            n152 = First Call?() -> (First Call?: T/F=w270:bool)
            n153 = control-ref of="Tree"() -> (w271:refnum<vi>)
            n154 = Select(t=w269, s=w270, f=string[] []) -> (s? t:f=w267:string[])
            n155 = call <vilib>:"NT Read and Format Entries as Tree.vi"("Tags to  Close"=w267, "Tree Refnum"=w271) -> ()  [unwired: 8 in, 2 out]
          }
          frame "Commands" {
            w280 = u32 5789784 ("Color Box")
            w281 = T26 {"Row"=-1, "Column"=-2} ("Active Cell:Active Cell")
            w283 = T26 {"Row"=-2, "Column"=-2} ("Active Cell:Active Cell")
            n156 = Index Array(array=w284, index=w278) -> (element=w282:u32)
            n157 = Index Array(array=w279, index=w278) -> (element=w277:T25)
            n158 = Unbundle(w277) -> ("Operation"=w276:enum16{"Update", "Clear"})  [unwired: 1 out]
            n159 = local read "Command Selection"() -> (w275:i32)
            n160 = property on="Command Selection" class="MCListbox (strict)"("ActiveCell"=w283, "CellBG"=w282, "ActiveCell"=w281, "CellBG"=w280) -> ()  [unwired: 2 in, 2 out]
            n161 = call <vilib>:"WPI_DashboardUpdate RPC Info.vi"("Operation"=w276) -> ("update"=w274:bool, "commands"=w273:string[][])  [unwired: 9 in]
            n162 = property on="Command Selection" class="MCListbox (strict)"("ItemNames"=w273) -> ()  [unwired: 2 in, 2 out]
            n163 = property on="Command Params" class="Tbl (strict)"("Active Cell"=w283, "Cell BG Color"=w282, "Active Cell"=w281, "Cell BG Color"=w280) -> ()  [unwired: 2 in, 2 out]
            n164 = call <vilib>:"WPI_DashboardUpdate Command Params.vi"("Update"=w274, "NewVal"=w275, "Commands"=w273, "Param Tbl"=w272) -> ()  [unwired: 7 in, 1 out]
          }
        }
        n165 = call <vilib>:"Connextion Info.vi"() -> ("Connected"=→"NT Connection":bool)  [unwired: 10 in, 1 out]
      }
      event "Test Tree": Value Change {
        # "Show appropriate\ncontrols"
        n166 = event-data() -> ("CtlRef"=w289:refnum<vi>, "NewVal"=w287:string)  [unwired: 1 in]
        n167 = call <vilib>:"WPI_UtilitiesGetTreeIOName.vi"("NewVal"=w287, "TreeControl in"=w289) -> ("I/O Name"=w290:string)  [unwired: 9 in]
        n168 = case shown="\"Camera\"" w290 {
          selector: w290 -> [_ w297 _ w319 w328 _]
          tunnel: w287 -> [_ _ w316 w318 _ w335]
          tunnel: cluster{string[]}[] [{["640x480", "320x240", "160x120"]}, {["Auto", "Fixed indoor", "Fixed outdoor 1", "Fixed outdoor 2", "Fixed fluorescent 1", "Fixed fluorescent 2", "Hold current"]}, {["Auto", "Flicker-free 50 Hz", "Flicker-free 60 Hz", "Hold current"]}, {["None", "Prioritize frame rate", "Prioritize image quality"]}, {["Monochrome", "Color"]}] -> [_ _ _ _ _ w334]
          frame Default {
            w292 = FALSE ("Visible")
            w291 = FALSE ("Visible")
            n169 = property on="Motor" class="Clust (strict)"("Visible"=w291) -> ()  [unwired: 2 in, 2 out]
            n170 = property on="Test Ring" class="Ring (strict)"("Visible"=w291) -> ()  [unwired: 2 in, 2 out]
            n171 = property on="Rev/Fwd" class="Clust (strict)"("Visible"=w292) -> ()  [unwired: 2 in, 2 out]
            n172 = property on="On/Off" class="Bool (strict)"("Visible"=w292) -> ()  [unwired: 2 in, 2 out]
            n173 = property on="Test Slider" class="Slide (strict)"("Visible"=w292) -> ()  [unwired: 2 in, 2 out]
          }
          frame "Analog Out", "Motor", "PWM" {
            w298 = FALSE ("Visible")
            n174 = case shown="\"Analog Out\"" w297 {
              tunnel: [1.0 ("Value") -1.0 ("Value") 0.0 ("Value")] -> w296
              tunnel: [255.0 ("Value") 1.0 ("Value") 5.0 ("Value")] -> w295
              tunnel: [128.0 ("Value") 0.0 ("Value") 0.0 ("Value")] -> w294
              tunnel: [64.0 ("Value") 0.5 ("Value") 1.0 ("Value")] -> w293
              frame "PWM" {
              }
              frame "Motor", Default {
              }
              frame "Analog Out" {
              }
            }
            n175 = property on="Motor" class="Clust (strict)"("Visible"=TRUE) -> ()  [unwired: 2 in, 2 out]
            n176 = property on="Value" class="Slide (strict)"("Value"=w294, "Scale.Minimum"=w296, "Scale.Maximum"=w295, "Scale.Increment"=w293) -> ()  [unwired: 2 in, 2 out]
            n177 = property on="On/Off" class="Bool (strict)"("Visible"=w298) -> ()  [unwired: 2 in, 2 out]
            n178 = property on="Test Slider" class="Slide (strict)"("Visible"=w298) -> ()  [unwired: 2 in, 2 out]
            n179 = property on="Test Ring" class="Ring (strict)"("Visible"=w298) -> ()  [unwired: 2 in, 2 out]
            n180 = property on="Rev/Fwd" class="Clust (strict)"("Visible"=w298) -> ()  [unwired: 2 in, 2 out]
          }
          frame "Servo" {
            w314 = FALSE ("Visible")
            n181 = call <vilib>:"NT Read Number.vi"("Name"=w316) -> ("Numeric"=w315:dbl)  [unwired: 9 in, 1 out]
            n182 = property on="Test Slider" class="Slide (strict)"("Visible"=TRUE, "Scale.Maximum"=170.0 ("Scale.Range:Maximum")) -> ()  [unwired: 2 in, 2 out]
            n183 = local write "Test Slider"(w315) -> ()
            n184 = property on="Motor" class="Clust (strict)"("Visible"=w314) -> ()  [unwired: 2 in, 2 out]
            n185 = property on="Rev/Fwd" class="Clust (strict)"("Visible"=w314) -> ()  [unwired: 2 in, 2 out]
            n186 = property on="On/Off" class="Bool (strict)"("Visible"=w314) -> ()  [unwired: 2 in, 2 out]
            n187 = property on="Test Ring" class="Ring (strict)"("Visible"=w314) -> ()  [unwired: 2 in, 2 out]
          }
          frame "Relay", "Solenoid" {
            w317 = FALSE ("Visible")
            n188 = property on="Motor" class="Clust (strict)"("Visible"=w317) -> ()  [unwired: 2 in, 2 out]
            n189 = property on="Test Slider" class="Slide (strict)"("Visible"=w317) -> ()  [unwired: 2 in, 2 out]
            n190 = Search and Replace String(input string=w318, search string="/Value  **", replace string="/Direction") -> (result string=w324:string)  [unwired: 5 in, 3 out]
            n191 = property on="Test Ring" class="Ring (strict)"("Visible"=w317) -> ()  [unwired: 2 in, 2 out]
            n192 = call <vilib>:"NT Read String.vi"("Name"=w324) -> ("String"=w322:string)  [unwired: 9 in, 1 out]
            n193 = Equal?(x="Both directions", y=w322) -> (x = y?=w320:bool)
            n194 = Not(x=w320) -> (.not. x?=w321:bool)
            n195 = property on="Rev/Fwd" class="Clust (strict)"("Visible"=w320) -> ()  [unwired: 2 in, 2 out]
            n196 = property on="On/Off" class="Bool (strict)"("Visible"=w321, "Caption.Text"=w319) -> ()  [unwired: 2 in, 2 out]
          }
          frame "Compressor", "Digital Out" {
            w327 = FALSE ("Visible")
            # "Get direction and finish"
            n197 = property on="Motor" class="Clust (strict)"("Visible"=w327) -> ()  [unwired: 2 in, 2 out]
            n198 = property on="Test Slider" class="Slide (strict)"("Visible"=w327) -> ()  [unwired: 2 in, 2 out]
            n199 = property on="Test Ring" class="Ring (strict)"("Visible"=w327) -> ()  [unwired: 2 in, 2 out]
            n200 = property on="On/Off" class="Bool (strict)"("Visible"=TRUE, "Caption.Text"=w328) -> ()  [unwired: 2 in, 2 out]
            n201 = property on="Rev/Fwd" class="Clust (strict)"("Visible"=FALSE) -> ()  [unwired: 2 in, 2 out]
          }
          frame "Camera" {
            n202 = call <vilib>:"Get Last Path Segment.vi"("String in"=w335) -> ("String out"=w336:string)  [unwired: 10 in]
            n203 = property on="On/Off" class="Bool (strict)"("Visible"=FALSE) -> ()  [unwired: 2 in, 2 out]
            n204 = property on="Motor" class="Clust (strict)"("Visible"=FALSE) -> ()  [unwired: 2 in, 2 out]
            n205 = property on="Rev/Fwd" class="Clust (strict)"("Visible"=FALSE) -> ()  [unwired: 2 in, 2 out]
            n206 = case shown="\"White Balance  **\"" w336 {
              tunnel: w335 -> [w342 w351 w360 w369 w378 _ w384]
              tunnel: w334 -> [w340 w348 w357 w366 w375 _ _]
              frame "Size  **" {
                n207 = Index Array(array=w340) -> (element=w339:cluster{string[]})  [unwired: 1 in]
                n208 = call <vilib>:"NT Read String.vi"("Name"=w342) -> ("String"=w341:string)  [unwired: 9 in, 1 out]
                n209 = Unbundle(w339) -> (w337:string[])
                n210 = Match First String(2:w337, 3:w341) -> (0:w338:i32)  [unwired: 1 out]
                n211 = property on="Test Ring" class="Ring (strict)"("Value"=w338, "Strings []"=w337) -> ()  [unwired: 2 in, 2 out]
                n212 = property on="Test Ring" class="Ring (strict)"("Visible"=TRUE) -> ()  [unwired: 2 in, 2 out]
                n213 = property on="Test Slider" class="Slide (strict)"("Visible"=FALSE) -> ()  [unwired: 2 in, 2 out]
              }
              frame "White Balance  **" {
                n214 = Index Array(array=w348, index=1) -> (element=w349:cluster{string[]})
                n215 = call <vilib>:"NT Read String.vi"("Name"=w351) -> ("String"=w350:string)  [unwired: 9 in, 1 out]
                n216 = Unbundle(w349) -> (w346:string[])
                n217 = Match First String(2:w346, 3:w350) -> (0:w345:i32)  [unwired: 1 out]
                n218 = property on="Test Ring" class="Ring (strict)"("Value"=w345, "Strings []"=w346) -> ()  [unwired: 2 in, 2 out]
                n219 = property on="Test Ring" class="Ring (strict)"("Visible"=TRUE) -> ()  [unwired: 2 in, 2 out]
                n220 = property on="Test Slider" class="Slide (strict)"("Visible"=FALSE) -> ()  [unwired: 2 in, 2 out]
              }
              frame "Exposure  **" {
                n221 = Index Array(array=w357, index=2) -> (element=w358:cluster{string[]})
                n222 = call <vilib>:"NT Read String.vi"("Name"=w360) -> ("String"=w359:string)  [unwired: 9 in, 1 out]
                n223 = Unbundle(w358) -> (w354:string[])
                n224 = Match First String(2:w354, 3:w359) -> (0:w355:i32)  [unwired: 1 out]
                n225 = property on="Test Ring" class="Ring (strict)"("Value"=w355, "Strings []"=w354) -> ()  [unwired: 2 in, 2 out]
                n226 = property on="Test Ring" class="Ring (strict)"("Visible"=TRUE) -> ()  [unwired: 2 in, 2 out]
                n227 = property on="Test Slider" class="Slide (strict)"("Visible"=FALSE) -> ()  [unwired: 2 in, 2 out]
              }
              frame "Exposure Priority  **" {
                n228 = Index Array(array=w366, index=3) -> (element=w367:cluster{string[]})
                n229 = call <vilib>:"NT Read String.vi"("Name"=w369) -> ("String"=w368:string)  [unwired: 9 in, 1 out]
                n230 = Unbundle(w367) -> (w363:string[])
                n231 = Match First String(2:w363, 3:w368) -> (0:w364:i32)  [unwired: 1 out]
                n232 = property on="Test Ring" class="Ring (strict)"("Value"=w364, "Strings []"=w363) -> ()  [unwired: 2 in, 2 out]
                n233 = property on="Test Ring" class="Ring (strict)"("Visible"=TRUE) -> ()  [unwired: 2 in, 2 out]
                n234 = property on="Test Slider" class="Slide (strict)"("Visible"=FALSE) -> ()  [unwired: 2 in, 2 out]
              }
              frame "Color Enable  **" {
                n235 = Index Array(array=w375, index=4) -> (element=w376:cluster{string[]})
                n236 = call <vilib>:"NT Read String.vi"("Name"=w378) -> ("String"=w377:string)  [unwired: 9 in, 1 out]
                n237 = Unbundle(w376) -> (w372:string[])
                n238 = Match First String(2:w372, 3:w377) -> (0:w373:i32)  [unwired: 1 out]
                n239 = property on="Test Ring" class="Ring (strict)"("Value"=w373, "Strings []"=w372) -> ()  [unwired: 2 in, 2 out]
                n240 = property on="Test Ring" class="Ring (strict)"("Visible"=TRUE) -> ()  [unwired: 2 in, 2 out]
                n241 = property on="Test Slider" class="Slide (strict)"("Visible"=FALSE) -> ()  [unwired: 2 in, 2 out]
              }
              frame Default {
                n242 = property on="Test Ring" class="Ring (strict)"("Visible"=FALSE) -> ()  [unwired: 2 in, 2 out]
                n243 = property on="Test Slider" class="Slide (strict)"("Visible"=FALSE) -> ()  [unwired: 2 in, 2 out]
              }
              frame "Brightness  **", "Color Level  **", "Compression  **", "FPS  **", "Sharpness  **" {
                n244 = call <vilib>:"NT Read Number.vi"("Name"=w384) -> ("Numeric"=w383:dbl)  [unwired: 9 in, 1 out]
                n245 = local write "Test Slider"(w383) -> ()
                n246 = property on="Test Slider" class="Slide (strict)"("Visible"=TRUE, "Scale.Maximum"=100.0 ("Scale.Range:Maximum")) -> ()  [unwired: 2 in, 2 out]
                n247 = property on="Test Ring" class="Ring (strict)"("Visible"=FALSE) -> ()  [unwired: 2 in, 2 out]
              }
            }
          }
        }
        n248 = property on="Progress" class="Clust (strict)"("Visible"=FALSE) -> ()  [unwired: 2 in, 2 out]
      }
      event "Test Name": Mouse Enter {
        # "Populate the ring with the list of tests"
        n249 = event-data() -> ()  [unwired: 1 in, 1 out]
        n250 = call <vilib>:"NT Read String Array.vi"("Name"="TestMode/TestList") -> ("String Array"=w392:string[])  [unwired: 9 in, 1 out]
        n251 = Build Array (concatenate)("Select the test to run...", w392) -> (w391:string[])
        n252 = property on="Test Name" class="Ring (strict)"("Strings []"=w391) -> ()  [unwired: 2 in, 2 out]
      }
      event "Test Name": Value Change {
        w394 = FALSE ("Visible")
        # "Tell the robot the test name to run"
        n253 = event-data() -> ("NewVal"=w398:u16)  [unwired: 1 in]
        n254 = property on="Test Name" class="Ring (strict)"() -> ("Strings []"=w399:string[])  [unwired: 2 in, 2 out]
        n255 = local write "Progress"(T5 {"Test Progress"=0, "Test Progress Text"=""} ("Progress")) -> ()
        n256 = Index Array(array=w399, index=w398) -> (element=w397:string)
        n257 = call <vilib>:"NT Write String.vi"("String"=w397, "Name"="TestMode/TestName") -> ()  [unwired: 9 in, 1 out]
        n258 = property on="Progress" class="Clust (strict)"("Visible"=TRUE) -> ()  [unwired: 2 in, 2 out]
        n259 = property on="Motor" class="Clust (strict)"("Visible"=w394) -> ()  [unwired: 2 in, 2 out]
        n260 = property on="Test Slider" class="Slide (strict)"("Visible"=w394) -> ()  [unwired: 2 in, 2 out]
        n261 = property on="On/Off" class="Bool (strict)"("Visible"=w394) -> ()  [unwired: 2 in, 2 out]
        n262 = property on="Rev/Fwd" class="Clust (strict)"("Visible"=w394) -> ()  [unwired: 2 in, 2 out]
        n263 = property on="Test Ring" class="Ring (strict)"("Visible"=w394) -> ()  [unwired: 2 in, 2 out]
      }
      event "Command Selection": Value Change {
        # "Get the params and show in table"
        n264 = event-data() -> ("NewVal"=w404:i32)  [unwired: 1 in]
        n265 = property on="Command Selection" class="MCListbox (strict)"() -> ("ItemNames"=w402:string[][])  [unwired: 2 in, 2 out]
        n266 = call <vilib>:"WPI_DashboardUpdate Command Params.vi"("NewVal"=w404, "Commands"=w402, "Param Tbl"=w403) -> ()  [unwired: 8 in, 1 out]
      }
      event "Execute Command": Value Change {
        # "Started one, Unique ID holds\nresponse"
        n267 = event-data() -> ()  [unwired: 1 in, 1 out]
        n268 = property on="Command Selection" class="MCListbox (strict)"() -> ("ItemNames"=w415:string[][])  [unwired: 2 in, 2 out]
        n269 = Index Array(array=w415, index (row)="Command Selection", index (col)=0) -> (element=w413:string)
        n270 = call <vilib>:"Invoke Commands.vi"("Command Params"="Command Params", "Function Name"=w413) -> ("Params"=w409:u8, "Started"=w408:bool)  [unwired: 7 in, 1 out]
        n271 = Array Subset(array="Command Params", length (row)=w409) -> (w410:string[][])  [unwired: 3 in]
        n272 = Select(t="Executing" ("Cmd Status"), s=w408, f="" ("Cmd Status")) -> (s? t:f=→"Cmd Status":string)
      }
      event "Command Selection": Double Click {
        n273 = event-data() -> ("Row"=w423:i32)  [unwired: 1 in]
        n274 = property on="Command Selection" class="MCListbox (strict)"() -> ("ItemNames"=w426:string[][])  [unwired: 2 in, 2 out]
        n275 = local read "Command Params"() -> (w422:string[][])
        n276 = Index Array(array=w426, index (row)=w423, index (col)=0) -> (element=w424:string)
        n277 = call <vilib>:"Invoke Commands.vi"("Command Params"=w422, "Function Name"=w424) -> ("Params"=w421:u8, "Started"=w416:bool)  [unwired: 7 in, 1 out]
        n278 = Array Subset(array=w422, length (row)=w421) -> (w420:string[][])  [unwired: 3 in]
        n279 = Select(t="Executing" ("Cmd Status"), s=w416, f="" ("Cmd Status")) -> (s? t:f=w417:string)
        n280 = local write "Cmd Status"(w417) -> ()
      }
      event "CheckList": Double Click {
        # "Shift clears all"
        # "Update symbols on the listbox"
        n281 = event-data() -> ("PlatMods.Shift"=w428:bool, "Row"=w430:i32)  [unwired: 1 in]
        n282 = case shown="True" w428 {
          tunnel: w430 -> [w434 _]
          tunnel: 1 -> [w433 _]
          frame False {
            n283 = property on="CheckList" class="LstBox (strict)"() -> ("Item Symbols"=w432:i32[])  [unwired: 2 in, 2 out]
            n284 = Replace Array Subset(array=w432, new element=w433, index=w434) -> (w431:i32[])
            n285 = property on="CheckList" class="LstBox (strict)"("Item Symbols"=w431) -> ()  [unwired: 2 in, 2 out]
          }
          frame True {
            w435 = 0 ("Top Row")
            n286 = property on="CheckList" class="LstBox (strict)"() -> ("Number of Rows"=w437:u32)  [unwired: 2 in, 2 out]
            n287 = Initialize Array(0, w437) -> (w436:i32[])
            n288 = property on="CheckList" class="LstBox (strict)"("Top Row"=w435, "Value"=w435, "Item Symbols"=w436) -> ()  [unwired: 2 in, 2 out]
          }
        }
      }
      event "CheckList": Key Down {
        # "Update symbols on the listbox\nLeft and right keys check and uncheck"
        n289 = event-data() -> ("VKey"=w441:T23)  [unwired: 1 in]
        n290 = case shown="\"Left\", \"Right\"" w441 {
          selector: w441 -> [w446 _]
          tunnel: eventvkey."Left" ("VKey") -> [w444 _]
          frame "Left", "Right" {
            n291 = Equal?(x=w444, y=w446) -> (x = y?=w445:bool)
            n292 = Select(t=0, s=w445, f=1) -> (s? t:f=w447:i32)
            n293 = property on="CheckList" class="LstBox (strict)"() -> ("Item Symbols"=w450:i32[])  [unwired: 2 in, 2 out]
            n294 = Replace Array Subset(array=w450, new element=w447, index="CheckList") -> (w449:i32[])
            n295 = property on="CheckList" class="LstBox (strict)"("Item Symbols"=w449) -> ()  [unwired: 2 in, 2 out]
          }
          frame Default {
          }
        }
      }
      event "Motor.Enable": Value Change {
        # "When the test mode otor enable helper is set, update that\ntree row item's value"
        n296 = event-data() -> ("NewVal"=w456:bool)  [unwired: 1 in]
        n297 = Unbundle("Motor") -> ("Value"=w455:dbl)  [unwired: 1 out]
        n298 = Select(t=w455, s=w456, f=0.0) -> (s? t:f=w453:dbl)
        n299 = call <vilib>:"NT Write Number.vi"("Numeric"=w453, "Name"=w452) -> ()  [unwired: 9 in, 1 out]
      }
      event "Test Slider": Value Change {
        # "When the test mode slider helper is set, update that\ntree row item's value"
        n300 = event-data() -> ("NewVal"=w459:dbl)  [unwired: 1 in]
        n301 = call <vilib>:"NT Write Number.vi"("Numeric"=w459, "Name"=w460) -> ()  [unwired: 9 in, 1 out]
      }
      event "On/Off": Value Change {
        # "When the test mode on/off helper value is set, update that\ntree row item's value"
        n302 = event-data() -> ("NewVal"=w464:bool)  [unwired: 1 in]
        n303 = Boolean To (0,1)(Boolean=w464) -> (0, 1=w463:i16)
        n304 = call <vilib>:"NT Write Number.vi"("Numeric"=w463, "Name"=w462) -> ()  [unwired: 9 in, 1 out]
      }
      event "Rev/Fwd": Value Change {
        # "When the test mode helper value for relays is set, update that\ntree row item's value"
        n305 = event-data() -> ("NewVal.Forward"=w472:bool, "NewVal.Reverse"=w471:bool)  [unwired: 1 in]
        n306 = Boolean To (0,1)(Boolean=w472) -> (0, 1=w468:i16)
        n307 = Boolean To (0,1)(Boolean=w471) -> (0, 1=w470:i16)
        n308 = Negate(x=w470) -> (-x=w469:i16)
        n309 = Add(x=w468, y=w469) -> (x+y=w467:i16)
        n310 = call <vilib>:"NT Write Number.vi"("Numeric"=w467, "Name"=w466) -> ()  [unwired: 9 in, 1 out]
      }
      event "Test Ring": Value Change {
        # "When a test mode helper value is selected from the ring,\nset the tree item's variable to the string value"
        n311 = event-data() -> ("NewVal"=w476:u16)  [unwired: 1 in]
        n312 = property on="Test Ring" class="Ring (strict)"() -> ("Strings []"=w477:string[])  [unwired: 2 in, 2 out]
        n313 = Index Array(array=w477, index=w476) -> (element=w475:string)
        n314 = call <vilib>:"NT Write String.vi"("String"=w475, "Name"=w474) -> ()  [unwired: 9 in, 1 out]
      }
      event "Rec Mode": Value Change {
        # "Update globals for recording mode and path to read log from.\nClear when logging and let NetworkTables set path for vision to\nuse."
        n315 = event-data() -> ("NewVal"=w488:enum32{"Stop", "Record", "Playback"})  [unwired: 1 in]
        n316 = global write "WPI_DashboardLogging Global.vi" "Logging Filename"(path "") -> ()
        n317 = global write "WPI_DashboardLogging Global.vi" "Recording"(w488) -> ()
        n318 = case shown="\"Playback\"" w488 {
          tunnel: w487 -> [_ w490 w499]
          tunnel: [_ _ w498] -> w485
          tunnel: [_ _ w497] -> _
          tunnel: w483 -> [_ _ w495]
          tunnel: cluster{i32, i32} {-250, 170} -> [_ _ w494]
          tunnel: [_ _ T24 {"Image Size"=TRUE, "Image Type"=TRUE, "Pixel Value"=TRUE, "ROI Information"=TRUE, "Zoom Factor"=FALSE} ("Image Information Shown:All Elements")] -> w478
          tunnel: [_ _ TRUE ("Zoom Factor")] -> w479
          tunnel: w481 -> [_ _ w491]
          frame Default {
          }
          frame "Stop", "Record" {
            # "Place Window too"
            n319 = invoke class="VI" method="FP.Close"(reference=w490) -> (reference out=w489:refnum<vi>)  [unwired: 2 in, 2 out]
            n320 = invoke class="VI" method="Abort VI"(reference=w489) -> ()  [unwired: 2 in, 3 out]
          }
          frame "Playback" {
            n321 = call "Open Playback Panel.vi"("Offset"=w494, "DB VI Ref"=w495, "Playback in"=w499) -> ("Playback out"=w496:refnum<vi>)  [unwired: 8 in]
            n322 = register-events(w496, w491) -> (reference out=w498:refnum<event-registration>, error out=w497:errorcluster)  [unwired: 2 in]
          }
        }
        n323 = property on="Camera Image Right" class="ImageControl"("Image Information Shown"=w478, "Image Information Visible"=w479) -> ()  [unwired: 2 in, 2 out]
        n324 = property on="Camera Image" class="ImageControl"("Image Information Shown"=w478, "Image Information Visible"=w479) -> ()  [unwired: 2 in, 2 out]
        n325 = call <vilib>:"WPI_DashboardNT Log FieldName Cache.vi"("Operation"=enum16{"Lookup/Add", "Index", "Clear"}."Clear") -> ()  [unwired: 8 in, 3 out]
      }
      event Panel Close {
        w501 = enum32{"Stop", "Record", "Playback"}."Stop" ("Rec Mode")
        # "Playback window has been closed, abort"
        n326 = event-data() -> ()  [unwired: 1 in, 4 out]
        n327 = local write "Rec Mode"(w501) -> ()
        n328 = global write "WPI_DashboardLogging Global.vi" "Recording"(w501) -> ()
      }
      event Panel Close {
        # "Abort playback window and ourself"
        n329 = event-data() -> ()  [unwired: 1 in, 4 out]
        n330 = invoke class="VI" method="FP.Close"(reference=w505) -> (reference out=w504:refnum<vi>)  [unwired: 2 in, 2 out]
        n331 = invoke class="VI" method="Abort VI"(reference=w504) -> (error out=w503:errorcluster)  [unwired: 2 in, 2 out]
        n332 = invoke class="VI" method="Abort VI"(error in=w503) -> ()  [unwired: 2 in, 3 out]
      }
      event User Event {
        n333 = event-data() -> ("IDs"=w512:cluster{"RPC field ID":u16, "Unique ID":u16}, "String"=w511:string)  [unwired: 1 in]
        n334 = Bundle("IDs"=w512, "String"=w511) -> (w510:T9)  [unwired: 1 in]
        n335 = call <vilib>:"Retrieve RPC Response.vi"("RPC Response"=w510) -> ("Output"=w508:string[][])  [unwired: 10 in]
        n336 = Build Array (concatenate)(w506, w508) -> (w507:string[][])
        n337 = local write "Command Params"(w507) -> ()
        n338 = local write "Cmd Status"("" ("Cmd Status")) -> ()
      }
      event "Tree": Double Click {
        n339 = event-data() -> ("PlatMods"=w518:T27, "Tag"=w515:string)  [unwired: 1 in]
        n340 = Unbundle(w518) -> ("Shift"=w517:bool)  [unwired: 4 out]
        n341 = String Subset(string=w515, length (rest)=1 ("length (rest)")) -> (substring=w514:string)  [unwired: 1 in]
        n342 = Not(x=w517) -> (.not. x?=w516:bool)
        n343 = case shown="\"/\"" w514 {
          tunnel: w515 -> [_ w521]
          tunnel: w516 -> [_ w520]
          frame Default {
          }
          frame "/" {
            n344 = call <vilib>:"NT Update Persistence.vi"("Persistence"=w520, "Name"=w521) -> ()  [unwired: 9 in, 1 out]
          }
        }
      }
    }
  }
  n345 = property on="On/Off" class="Bool (strict)"("Visible"=w35) -> ()  [unwired: 2 in, 2 out]
  n346 = property on="Motor" class="Clust (strict)"("Visible"=w35) -> ()  [unwired: 2 in, 2 out]
  n347 = property on="Progress" class="Clust (strict)"("Visible"=w35) -> ()  [unwired: 2 in, 2 out]
  n348 = property on="Test Ring" class="Ring (strict)"("Visible"=w35) -> ()  [unwired: 2 in, 2 out]
  n349 = property on="Rev/Fwd" class="Clust (strict)"("Visible"=w35) -> ()  [unwired: 2 in, 2 out]
  n350 = local write "Command Selection"(u16 0 ("milliseconds to wait")) -> ()
  n351 = while {
    tunnel: u16 1741 ("timeout ms (25000)") -> [w523]
    stop <- FALSE stop-if-true
    n352 = TCP Create Listener(10:w523) -> (0:w522:errorcluster, 3:w524:refnum<k5>)  [unwired: 4 in, 1 out]
    n353 = case shown="No Error" w522 {
      selector: w522 -> [w526 _]
      tunnel: w524 -> [w527 _]
      frame No Error {
        n354 = while {
          tunnel: w527 -> [w530]
          tunnel: w526 -> [w529]
          stop <- FALSE stop-if-true
          n355 = TCP Wait On Listener(8:w529, 11:w530) -> (0:w531:errorcluster, 4:w532:refnum<k5>)  [unwired: 2 in, 3 out]
          n356 = local write "TCP"(w532) -> ()
          n357 = case shown="No Error" w531 {
            frame No Error {
            }
            frame Error {
              n358 = Wait (ms)(milliseconds to wait=u32 1000) -> ()  [unwired: 1 out]
            }
          }
        }
      }
      frame Error {
        n359 = Wait (ms)(milliseconds to wait=u32 1000) -> ()  [unwired: 1 out]
      }
    }
  }
  n360 = local write "Command Params"(string[][] [] ("Command Params")) -> ()
  n361 = global write "WPI_DashboardLogging Global.vi" "Recording"(w58) -> ()
  n362 = local write "Rec Mode"(w58) -> ()
  n363 = call <vilib>:"NT Write String.vi"("Name"="Auto Selector") -> ()  [unwired: 10 in, 1 out]
